vi "MultiChannel Write.vi"(8 "Error In":errorcluster, 10 "Data to Log":dbl[][](array[numeric]), 11 "File Refnum In":refnum<file>) -> (0 "Error Out":errorcluster, 3 "File Refnum Out":refnum<file>)   [LabVIEW 2017]
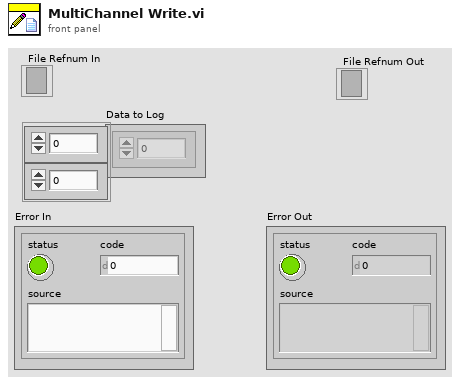
[diagram p1: front panel]
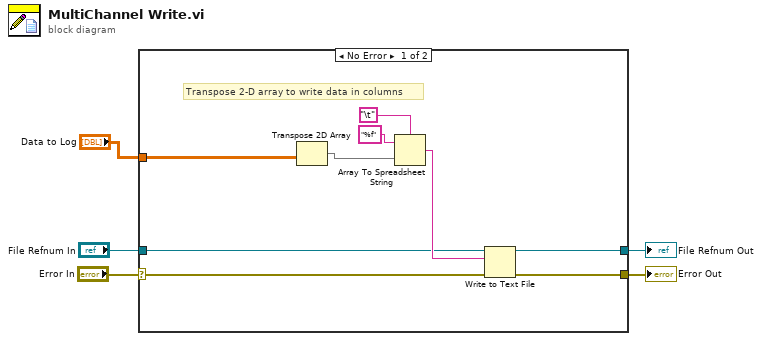
[diagram p0: block diagram]
diagram:
  n1 = case shown="No Error" "Error In" {
    selector: "Error In" -> [w7 w16]
    tunnel: "File Refnum In" -> [w9 w15]
    tunnel: [w8 w15] -> w3
    tunnel: [w6 w16] -> w2
    tunnel: "Data to Log" -> [w14 _]
    frame No Error {
      # "Transpose 2-D array to write data in columns"
      n2 = Transpose 2D Array(2D array=w14) -> (transposed array=w11:dbl[][])
      n3 = Array To Spreadsheet String(delimiter (Tab)="\t", array=w11, 3:"%f" ("format string")) -> (spreadsheet string=w10:string)
      n4 = Write to Text File(file (use dialog)=w9, text=w10, error in=w7) -> (refnum out=w8:refnum<file>, error out=w6:errorcluster)  [unwired: 1 in, 1 out]
    }
    frame Error {
    }
  }
  "Error Out" <- w2
  "File Refnum Out" <- w3
